vi "Add Element to Constant.vi"(9 "Element Name":string, 10 "Cluster or Array":refnum<vi>, 11 "Opaque Struct Writer in":refnum<class "Opaque Struct Writer.lvclass">) -> (2 "Cluster or Array Dup":refnum<vi>, 3 "Opaque Struct Writer out":refnum<class "Opaque Struct Writer.lvclass">)   [LabVIEW 2014, in "Opaque Struct Writer.lvclass"]
doc: "Copyright (c) 2016 Sze Howe Koh\n\nThis Source Code Form is subject to the terms of the Mozilla Public License, v. 2.0. If a copy of the MPL was not distributed with this file, You can obtain one at http://mozilla.org/MPL/2.0/."
uses:
  Opaque Struct Writer.lvclass
  String Writer/String Writer.lvclass
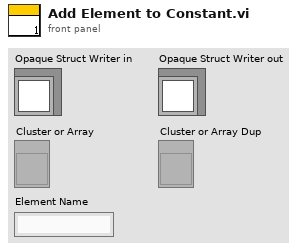
[diagram p1: front panel]
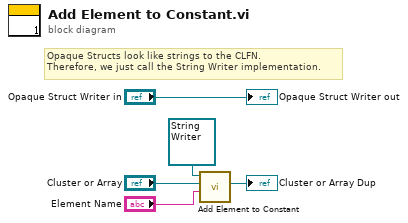
[diagram p0: block diagram]
diagram:
  # "Opaque Structs look like strings to the CLFN.\nTherefore, we just call the String Writer implementation."
  n1 = call-dynamic "Add Element to Constant.vi"("Element Name"="Element Name", "Cluster or Array"="Cluster or Array", "String Writer in"=refnum<class "String Writer.lvclass"> refnum) -> ("Cluster or Array Dup"=→"Cluster or Array Dup":refnum<vi>)  [unwired: 7 in, 1 out]
  "Opaque Struct Writer out" <- "Opaque Struct Writer in"
